vi "HostQueuesTest.vi"() -> ()   [LabVIEW 2014]
panel:
  out "Element number":u8(slide) scale=1.0..200.0
  in  "FastOut?":bool
  in  "FastIn?":bool
  in  "stop":bool
  out "Output Element":i32(graph)
  out "Input Element":dbl(graph)
  out "LastElement":i32
  out "# elements in queue":i32
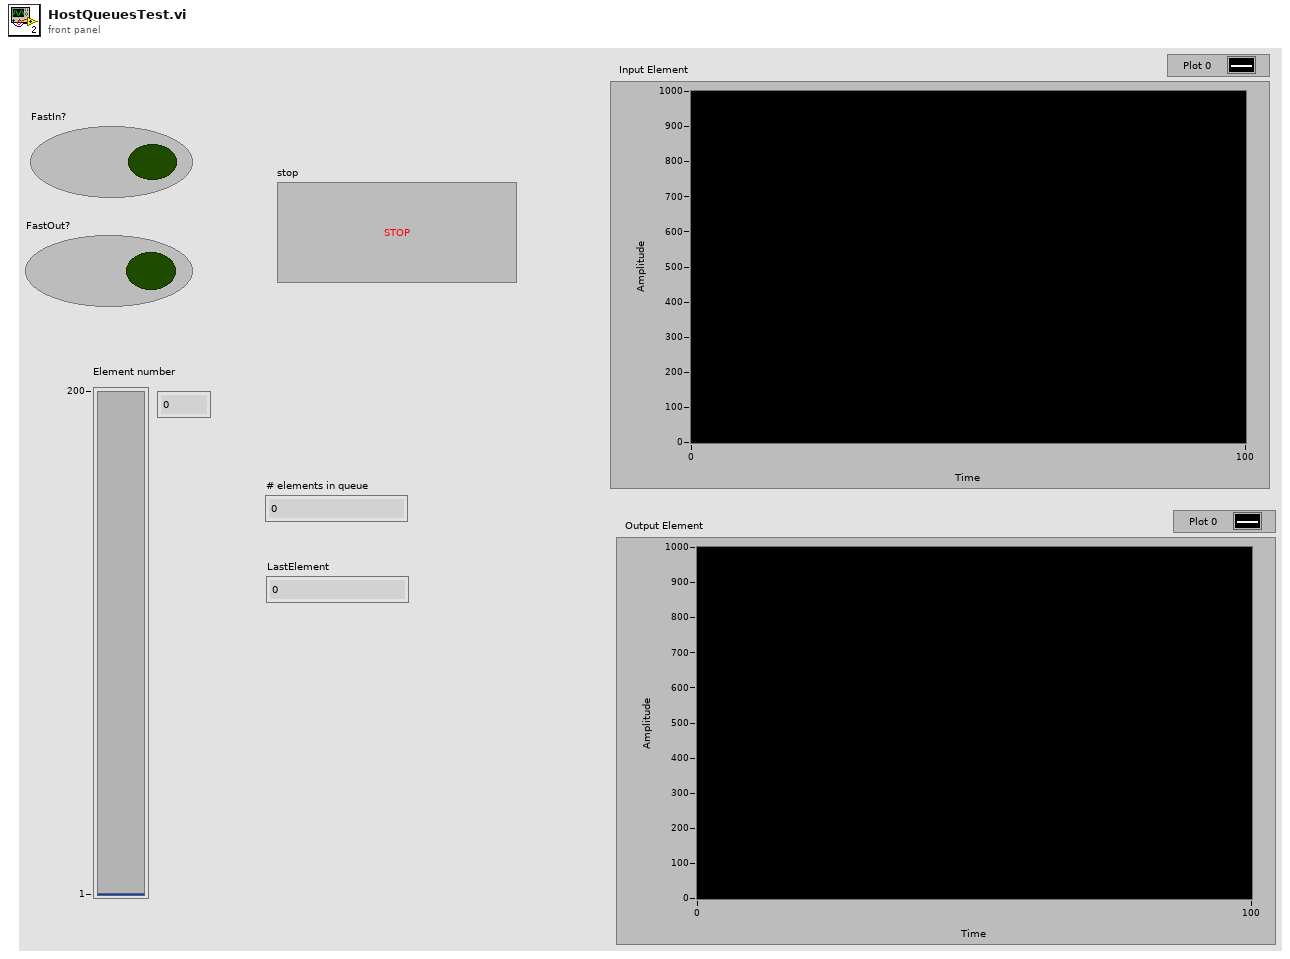
[diagram p1: front panel]
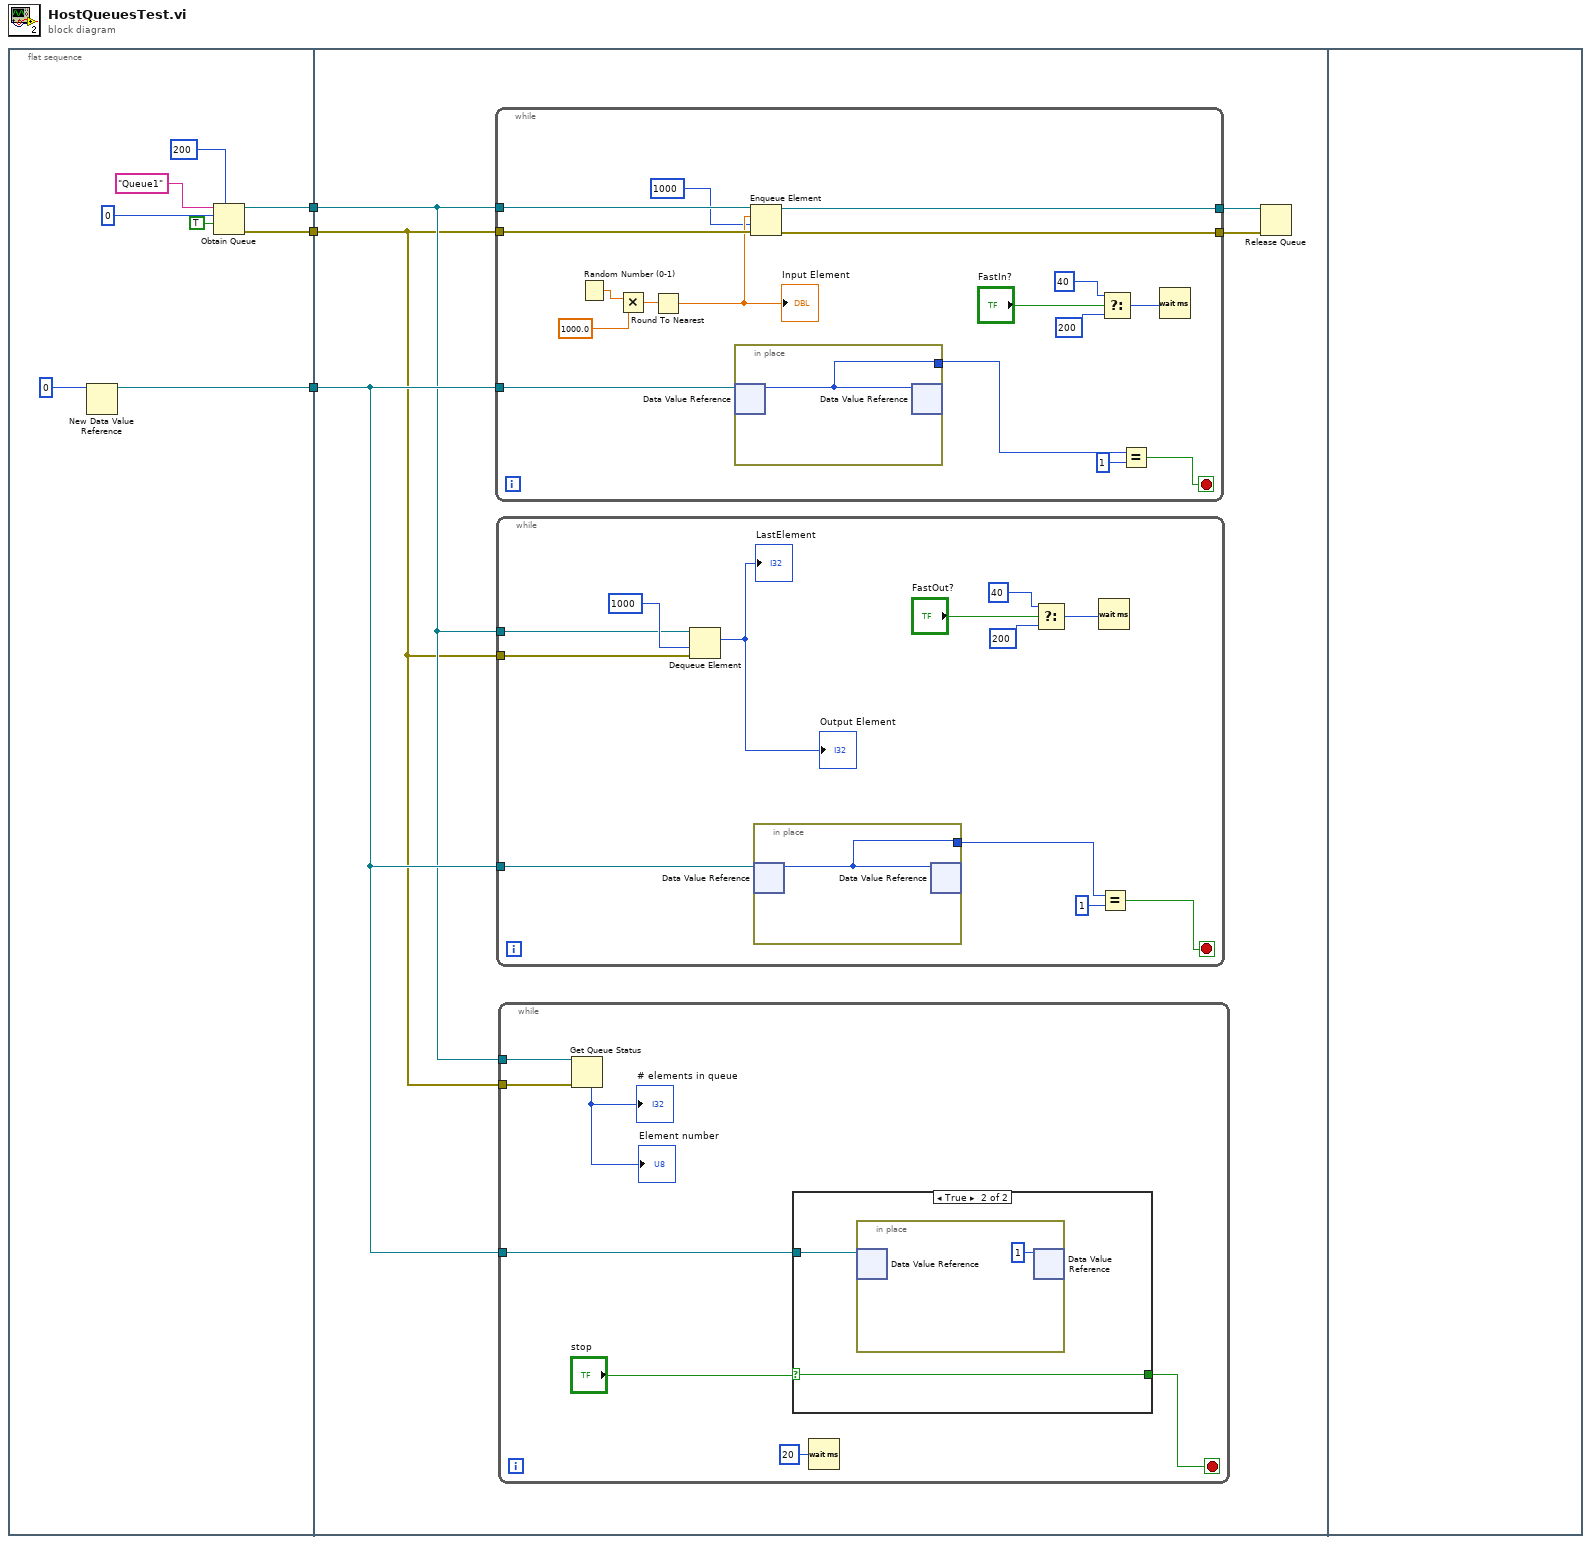
[diagram p0: block diagram]
diagram:
  n1 = flat-sequence {
    tunnel: [w8] -> w3
    tunnel: [w7] -> w2
    tunnel: [w4] -> w1
    tunnel: w3 -> [w13]
    tunnel: w2 -> [w12]
    tunnel: w1 -> [w14]
    frame #0 {
      n2 = New Data Value Reference(data value=0) -> (data value reference=w4:refnum<data-value>)  [unwired: 1 in, 1 out]
      n3 = Obtain Queue(max queue size (-1, unlimited)=200, name (unnamed)="Queue1", element data type=0, create if not found? (T)=TRUE) -> (queue out=w8:refnum<queue>, error out=w7:errorcluster)  [unwired: 1 in, 1 out]
    }
    frame #1 {
      n4 = while {
        tunnel: w13 -> [w57]
        tunnel: w12 -> [w56]
        tunnel: [w55] -> w16
        tunnel: [w50] -> w15
        tunnel: w14 -> [w48]
        stop <- w45 stop-if-true
        n5 = Random Number (0-1)() -> (number: 0 to 1=w54:dbl)
        n6 = Multiply(x=w54, y=1000.0) -> (x*y=w52:dbl)
        n7 = Round To Nearest(number=w52) -> (nearest integer value=w51:dbl)
        "Input Element" <- w51
        n8 = in-place {
          in-place-border: [w58] -> w47
          n9 = in-place-dvr #1(w48) -> (w58:i32)  [unwired: 1 out]
          n10 = in-place-dvr #1(w58) -> ()  [unwired: 2 out]
        }
        n11 = Enqueue Element(queue=w57, element=w51, timeout in ms (-1)=1000, error in (no error)=w56) -> (queue out=w55:refnum<queue>, error out=w50:errorcluster)  [unwired: 1 out]
        n12 = Select(t=40, s="FastIn?", f=200) -> (s? t:f=w41:i32)
        n13 = Equal?(x=w47, y=1) -> (x = y?=w45:bool)
        n14 = Wait (ms)(milliseconds to wait=w41) -> ()  [unwired: 1 out]
      }
      n15 = while {
        tunnel: w13 -> [w37]
        tunnel: w12 -> [w36]
        tunnel: w14 -> [w35]
        stop <- w32 stop-if-true
        n16 = Dequeue Element(queue=w37, timeout in ms (-1)=1000, error in (no error)=w36) -> (element=→"LastElement" →"Output Element":i32)  [unwired: 3 out]
        n17 = in-place {
          in-place-border: [w40] -> w33
          n18 = in-place-dvr #2(w35) -> (w40:i32)  [unwired: 1 out]
          n19 = in-place-dvr #2(w40) -> ()  [unwired: 2 out]
        }
        n20 = Select(t=40, s="FastOut?", f=200) -> (s? t:f=w28:i32)
        n21 = Wait (ms)(milliseconds to wait=w28) -> ()  [unwired: 1 out]
        n22 = Equal?(x=w33, y=1) -> (x = y?=w32:bool)
      }
      n23 = while {
        tunnel: w14 -> [w20]
        tunnel: w13 -> [w18]
        tunnel: w12 -> [w17]
        stop <- w21 stop-if-true
        n24 = Get Queue Status(queue=w18, error in (no error)=w17) -> (# elements in queue=→"# elements in queue" →"Element number":i32)  [unwired: 1 in, 7 out]
        n25 = case shown="True" "stop" {
          selector: "stop" -> [w24 w26]
          tunnel: [w24 w26] -> w21
          tunnel: w20 -> [_ w25]
          frame False {
          }
          frame True {
            n26 = in-place {
              n27 = in-place-dvr #3(w25) -> ()  [unwired: 2 out]
              n28 = in-place-dvr #3(1 ("data value")) -> ()  [unwired: 2 out]
            }
          }
        }
        n29 = Wait (ms)(milliseconds to wait=u32 20) -> ()  [unwired: 1 out]
      }
      n30 = Release Queue(queue=w16, error in (no error)=w15) -> ()  [unwired: 1 in, 3 out]
    }
    frame #2 {
    }
  }
